vi "MagEncoder_cal_v2.vi"() -> ()   [LabVIEW 2014]
uses:
  <vilib>/eio/EIONode/EIONode.xnode
  <vilib>/rvi/eio/common/nirviEmuTemplateMethod_errors.vi
  <vilib>/rvi/Analysis/measure/butterworth/XNode/niFpgaButterworthFilter.xnode
  <vilib>/rvi/DataTransferAndStorage/Container/XNode/niFpgaContainer.xnode
  <vilib>/rvi/FXPMathLib/FxpSinAndCos/XNode/nifxpmath_SinAndCos.xnode
  <vilib>/rvi/FXPMathLib/FxpSinAndCos/simVIs/DllFxpSinAndCosTemp_sub.vi
  <vilib>/rvi/FXPMathLib/FxpSinAndCos/subVIs/nifxpmath_SinAndCos_SimConfig.ctl
  <vilib>/rvi/interface/RandomDataEmulation/nirviRandomDataFpgaMultiElementTemplate.vi
panel:
  in  "Vy (mm/s)":fxp<+/-,30,6>
  out "Dyr_ramp":fxp<+/-,22,7>
  in  "Dyr_stroke":fxp<+/-,32,7>
  out "Dpr_ramp":fxp<+/-,22,7>
  in  "Dpr_stroke":fxp<+/-,32,7>
  in  "Vp (mm/s)":fxp<+/-,30,6>
  out "omega_p (Mavg w. f)":fxp<+/-,36,18>
  in  "scaled coefficients":i32[](array[numeric])=[946630756, 63555534]
  in  "FIFO":i16(ring) items=["Pitch_F+P", "Yaw_F+P"]
  out "PID (kHz)":fxp<+/-,20,10>
  in  "Set 6":bool
  in  "Set 5":bool
  in  "Set 4":bool
  in  "Set 3":bool
  in  "Set 2":bool
  in  "Set 1":bool
  out "Dy1_d (T)":fxp<+/-,36,13>
  out "omega_y1 (T)":fxp<+/-,36,13>
  out "Dp1_d (T)":fxp<+/-,36,13>
  out "omega_p1 (T)":fxp<+/-,36,13>
  out "Dy2_d (T)":fxp<+/-,36,13>
  out "Dp2_d (T)":fxp<+/-,36,13>
  out "omega_y2 (T)":fxp<+/-,36,13>
  out "omega_p2 (T)":fxp<+/-,36,13>
  out "mt_omega_y2":u32
  out "mt_omega_p2":u32
  out "rad_y2":fxp<+/-,33,20>
  out "D_y2":fxp<+/-,32,7>
  out "rad_y1":fxp<+/-,33,20>
  out "D_y1":fxp<+/-,32,7>
  out "Encoder Position_y1":i32
  out "Encoder Position_y2":i32
  out "Encoder Position_p2":i32
  out "D_p2":fxp<+/-,32,7>
  out "rad_p2":fxp<+/-,33,20>
  out "D_p1":fxp<+/-,32,7>
  out "rad_p1":fxp<+/-,33,20>
  out "Encoder Position_p1":i32
  in  "Mag. factor_y":fxp<+/-,20,3>
  in  "Mag. encoder_y":bool
  out "omega_y (rad/s)":fxp<+/-,36,13>
  out "Dy_d (mm/s)":fxp<+/-,36,13>
  in  "Vy. Est.":i16(ring) items=["T", "Mavg"]
  out "omega_y (Mavg)":fxp<+/-,36,14>
  out "Dy_d (Mavg)":fxp<+/-,36,14>
  in  "Dy_d_M_avg_Tc (uSec)":i32
  out "Dp_d (Mavg)":fxp<+/-,36,14>
  out "omega_p (Mavg)":fxp<+/-,36,14>
  in  "Dp_d_M_avg_Tc (uSec)":i32
  out "Dp_d (T)":fxp<+/-,36,13>
  out "omega_p (T)":fxp<+/-,36,13>
  in  "Vp. Est.":i16(ring) items=["T", "Mavg"]
  in  "Mag. factor_p":fxp<+/-,20,3>
  in  "Mag. encoder_p":bool
  in  "Belt_out_p":fxp<+/-,7,7>
  in  "Belt_in_p":fxp<+/-,6,6>
  in  "Belt_out_y":fxp<+/-,7,7>
  in  "Belt_in_y":fxp<+/-,6,6>
  in  "mt0_omega_p":u32
  in  "Encoder reset":bool
  out "Dpr_sin":fxp<+/-,22,7>
  in  "Sin offset_p":fxp<+/-,22,7>
  in  "Sin magnitude_p":fxp<+/-,21,6>
  out "Dpr_sin_dd":fxp<+/-,35,20>
  out "Dpr_sin_d":fxp<+/-,33,15>
  out "Sin omega_p":fxp<+/-,34,9>
  in  "Sin wave freq._p (Hz)":fxp<+/-,32,6>
  in  "Dpr_step":fxp<+/-,22,7>
  out "Dpr_for":fxp<+/-,22,7>
  in  "Command_p":i16(ring) items=["Step", "Sine", "Ramp"]
  out "Fp_PID":fxp<+/-,36,16>
  in  "Kp_p":fxp<+/-,32,13>
  out "va_p":fxp<+/-,36,7>
  out "vb_p":fxp<+/-,37,8>
  out "vq_p_F":fxp<+/-,20,5> format="%.57g"
  out "vd_p_F":fxp<+/-,20,5>
  in  "Stop motor_p":bool
  out "Dp_d (mm/s)":fxp<+/-,36,13>
  out "omega_p (rad/s)":fxp<+/-,36,13>
  out "mt_omega_p1":u32
  out "rad_p(NrTheta)":fxp<+/-,33,20>
  out "D_p(mm)":fxp<+/-,32,7>
  out "Encoder Position_p":i32
  in  "Encoder reset_p":bool
  out "Dyr_for":fxp<+/-,22,7>
  in  "Command_y":i16(ring) items=["Step", "Sine", "Ramp"]
  out "vb_y":fxp<+/-,38,8>
  out "va_y":fxp<+/-,38,8>
  out "Dyr_sin_dd":fxp<+/-,35,20>
  out "Dyr_sin_d":fxp<+/-,33,15>
  out "Sin omega_y":fxp<+/-,34,9>
  out "Dyr_sin":fxp<+/-,22,7>
  in  "Sin offset_y":fxp<+/-,22,7>
  in  "Sin magnitude_y":fxp<+/-,21,6>
  out "Time now(s)":fxp<+,52,14>
  in  "Sin wave freq._y (Hz)":fxp<+/-,32,6>
  in  "Dyr_step":fxp<+/-,22,7>
  out "Fy_PID":fxp<+/-,36,16>
  in  "Kp_y":fxp<+/-,32,13>
  out "vq_y_F":fxp<+/-,20,5> format="%.57g"
  out "vd_y_F":fxp<+/-,20,5>
  in  "Stop motor_y":bool
  out "Dy_d (T)":fxp<+/-,36,13>
  out "omega_y (T)":fxp<+/-,36,13>
  in  "mt0_omega_y":u32
  out "mt_omega_y1":u32
  out "rad_y(NrTheta)":fxp<+/-,33,20>
  out "D_y(mm)":fxp<+/-,32,7>
  out "Encoder Position_y":i32
  in  "Encoder reset_y":bool
  in  "Ini coe.":bool
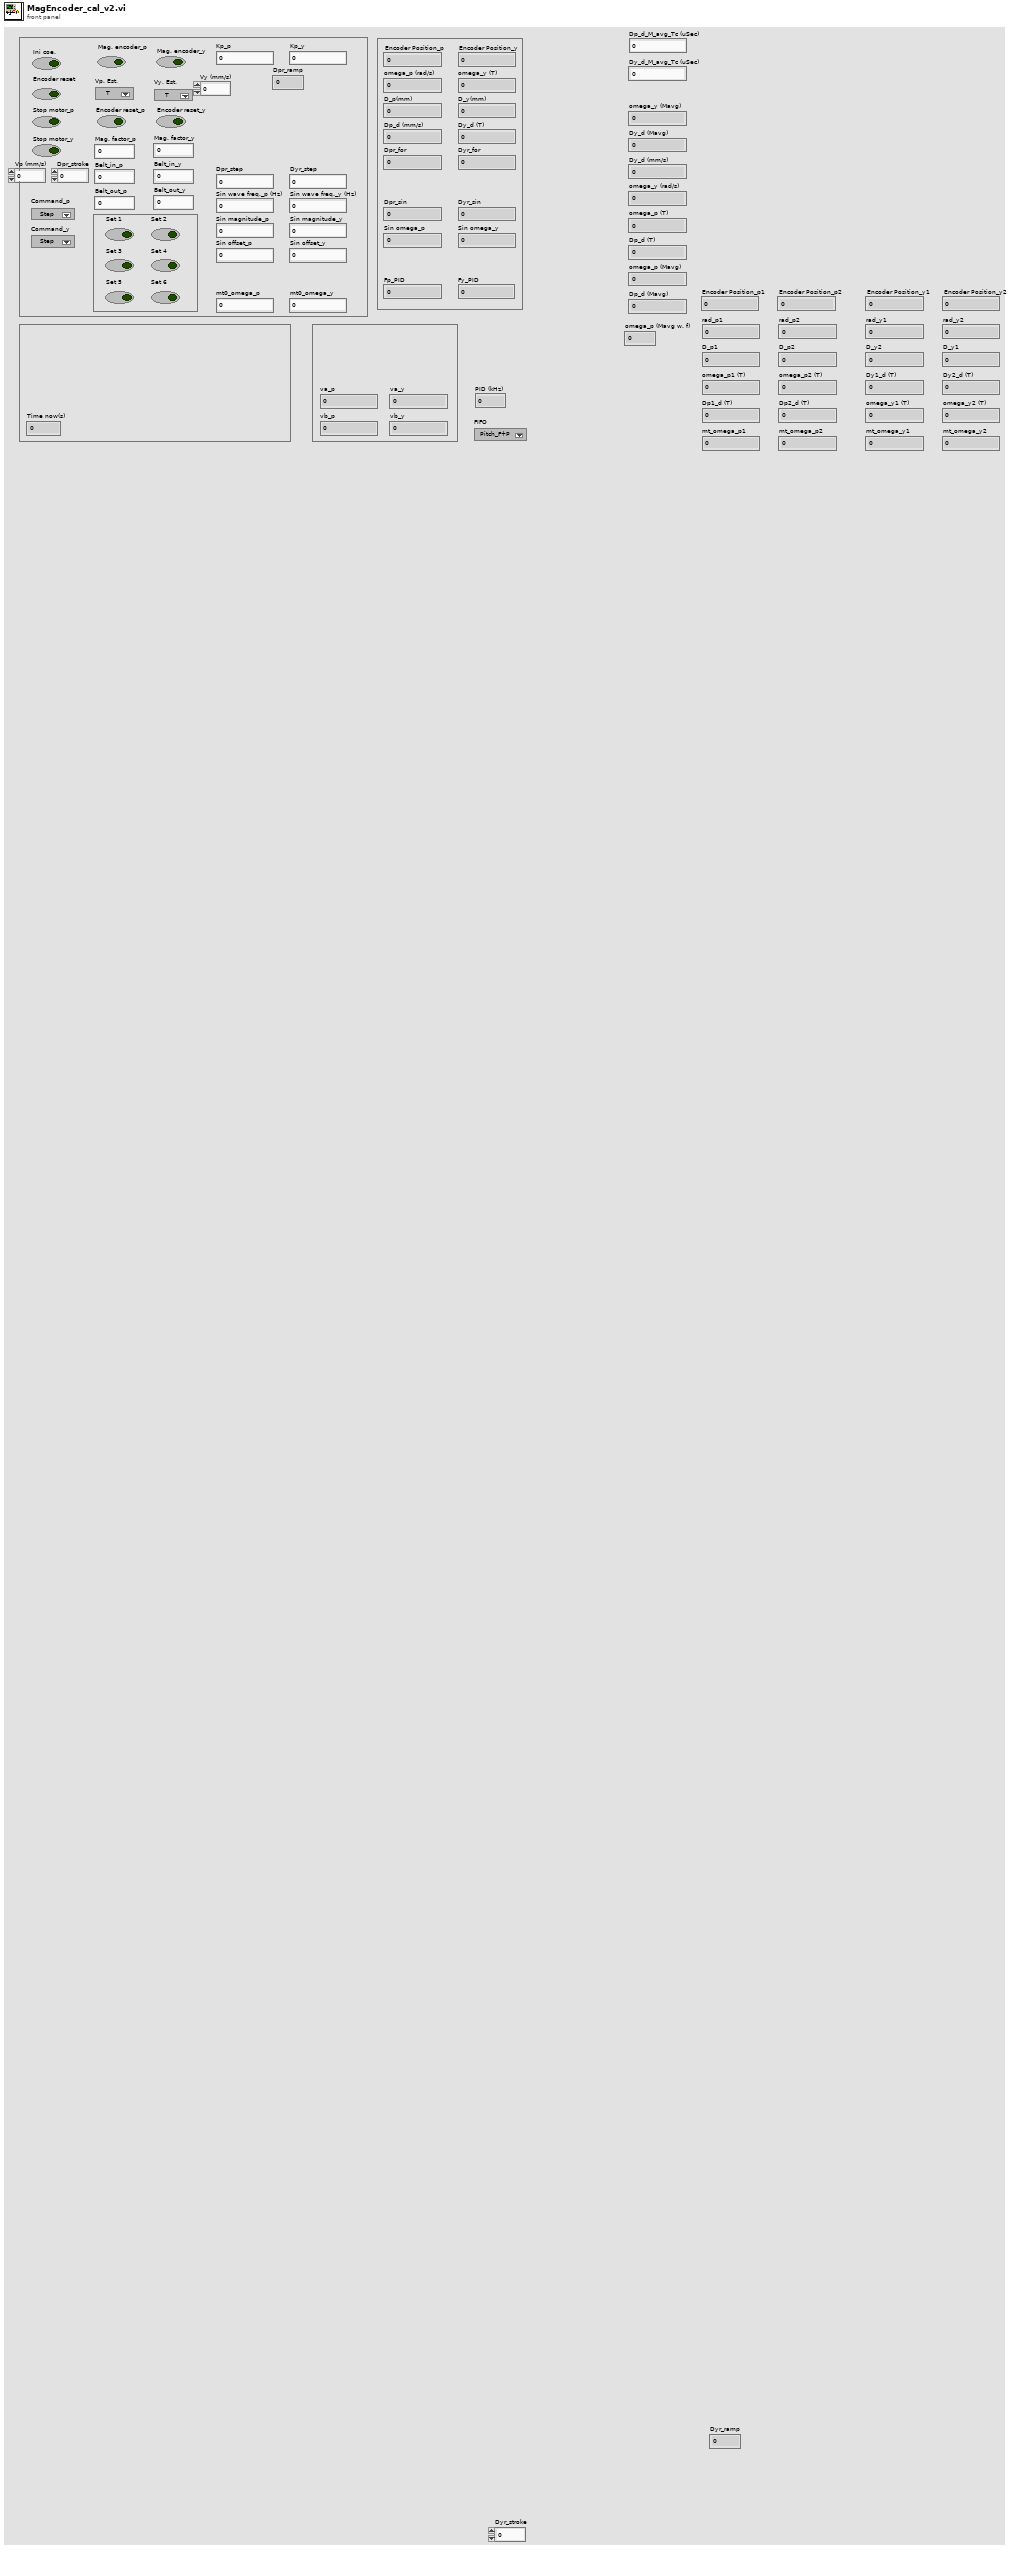
[diagram p1: front panel]
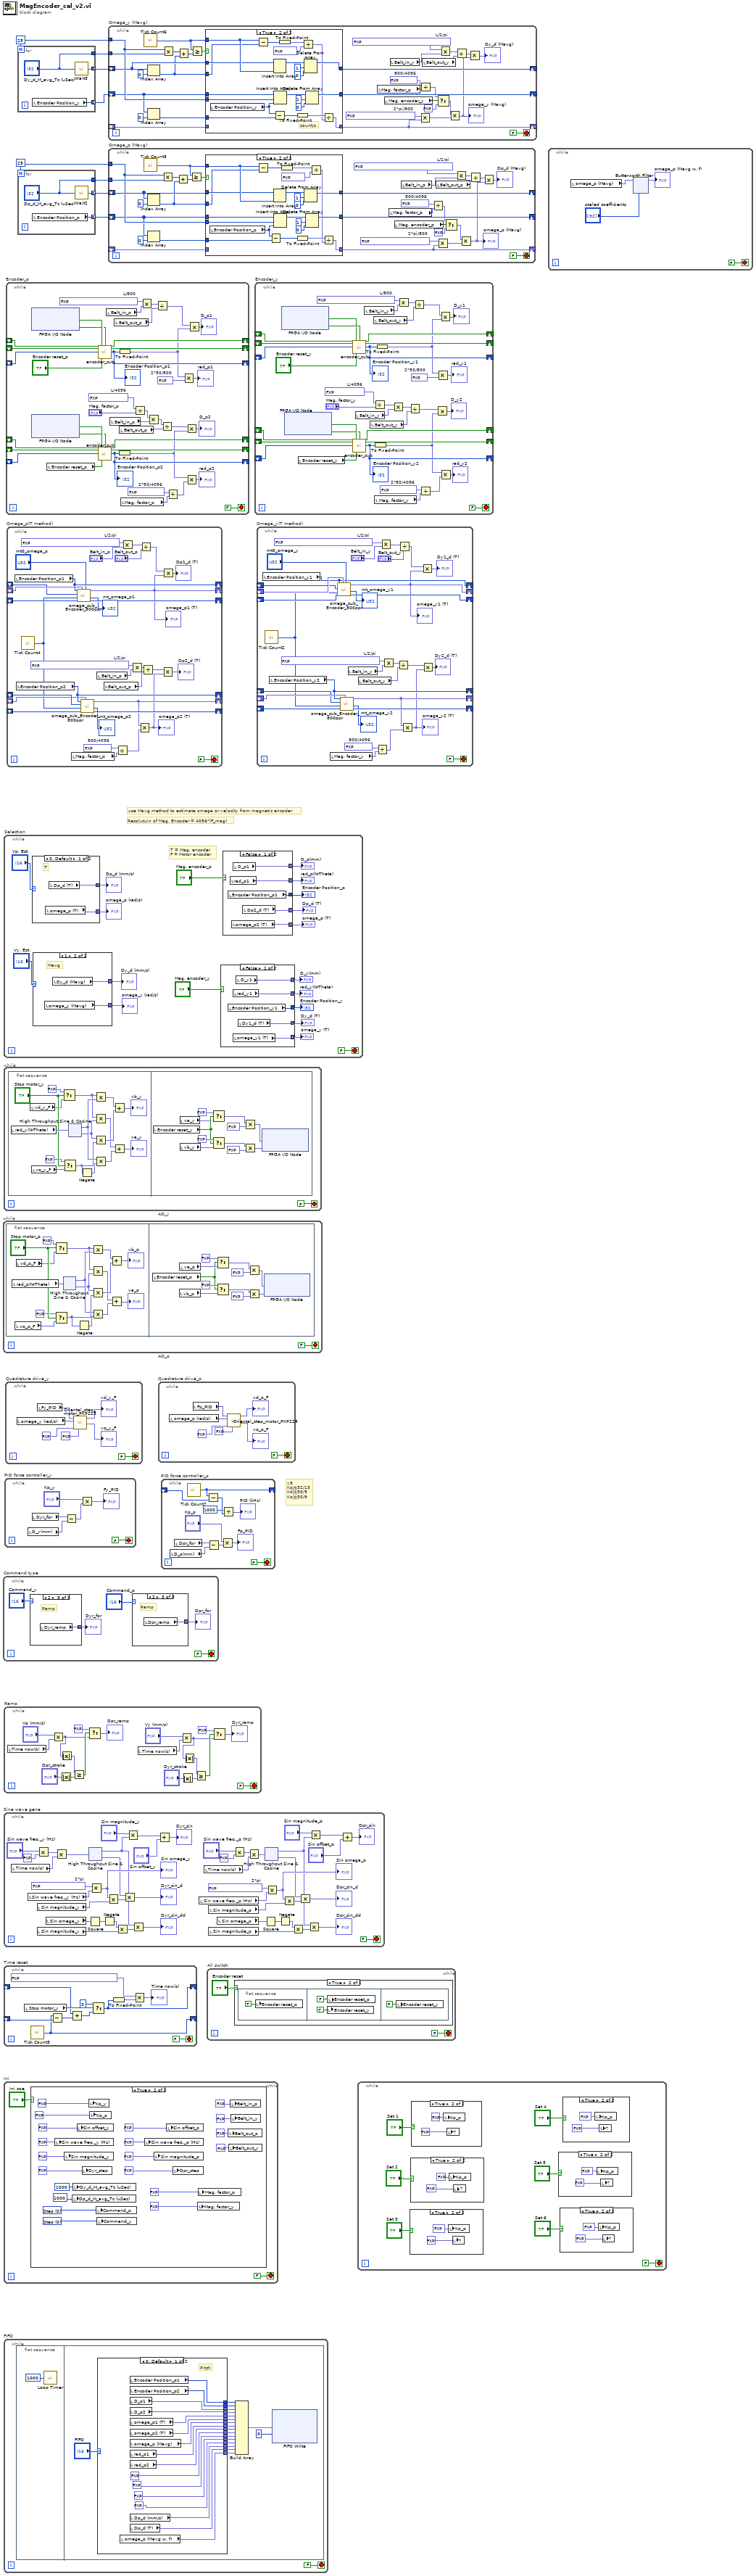
[diagram p0: block diagram]
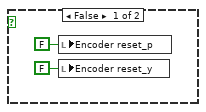
[diagram p10: hidden frame]
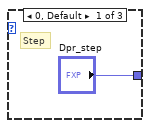
[diagram p11: hidden frame]
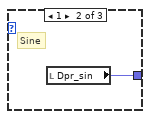
[diagram p12: hidden frame]
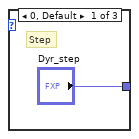
[diagram p13: hidden frame]
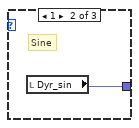
[diagram p14: hidden frame]
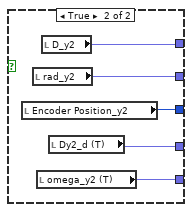
[diagram p15: hidden frame]
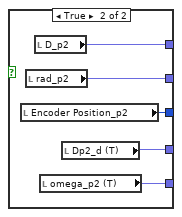
[diagram p16: hidden frame]
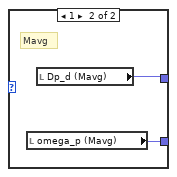
[diagram p17: hidden frame]
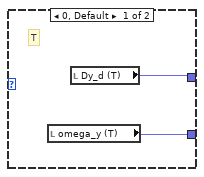
[diagram p18: hidden frame]
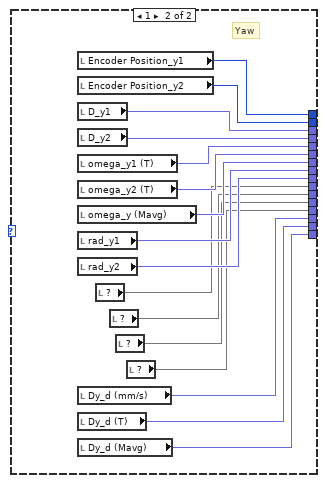
[diagram p20: hidden frame]
diagram:
  w5 = 25
  w8 = 25
  # "v9\nKp改32/13\nKd改30/9\nKo改30/9"
  # "Resolutuin of Mag. Encoder = 4096*(F_mag)"
  # "use Mavg method to estimate omega or velocity from magnetic encoder"
  n1 = while "AO_p" {
    stop <- FALSE stop-if-true
    n2 = flat-sequence {
      frame #0 {
        n3 = local read "rad_p(NrTheta)"() -> (w21:fxp<+/-,33,20>)
        n4 = local read "vq_p_F"() -> (w22:fxp<+/-,20,5>)
        n5 = local read "vd_p_F"() -> (w24:fxp<+/-,20,5>)
        n6 = Select(t=fxp<+/-,20,5> 0.0, s="Stop motor_p", f=w24) -> (s? t:f=w13:fxp<+/-,20,5>)
        n7 = Select(t=fxp<+,1,1> 0.0, s="Stop motor_p", f=w22) -> (s? t:f=w12:fxp<+/-,20,5>)
        n8 = xnode "High Throughput Sine & Cosine"("x (pi)"=w21) -> ("sin(x)"=w15:fxp<+/-,16,2>, "cos(x)"=w14:fxp<+/-,16,2>)
        n9 = Negate(x=w12) -> (-x=w20:fxp<+/-,21,6>)
        n10 = Multiply(x=w13, y=w15) -> (x*y=w19:fxp<+/-,36,7>)
        n11 = Multiply(x=w13, y=w14) -> (x*y=w17:fxp<+/-,36,7>)
        n12 = Multiply(x=w14, y=w12) -> (x*y=w18:fxp<+/-,36,7>)
        n13 = Multiply(x=w15, y=w20) -> (x*y=w16:fxp<+/-,35,6>)
        n14 = Add(x=w19, y=w18) -> (x+y=→"vb_p":fxp<+/-,37,8>)
        n15 = Add(x=w17, y=w16) -> (x+y=→"va_p":fxp<+/-,36,7>)
      }
      frame #1 {
        n16 = local read "Encoder reset_p"() -> (w57:bool)
        n17 = local read "vb_p"() -> (w58:fxp<+/-,37,8>)
        n18 = local read "va_p"() -> (w59:fxp<+/-,36,7>)
        n19 = Select(t=fxp<+,2,2> 3.0, s=w57, f=w59) -> (s? t:f=w65:fxp<+/-,36,7>)
        n20 = Select(t=fxp<+,1,1> 0.0, s=w57, f=w58) -> (s? t:f=w64:fxp<+/-,37,8>)
        n21 = Multiply(x=w65, y=fxp<+/-,1,0> -0.5) -> (x*y=w60:fxp<+/-,36,6>)
        n22 = Multiply(x=w64, y=fxp<+/-,1,0> -0.5) -> (x*y=w61:fxp<+/-,36,6>)
        n23 = xnode "FPGA I/O Node"("Mod8/AO0"=w60, "Mod8/AO1"=w61) -> ()  [unwired: 2 in, 2 out]
      }
    }
  }
  n24 = while "Command type" {
    stop <- FALSE stop-if-true
    n25 = case shown="2" "Command_y" {
      tunnel: ["Dyr_step" w77 w78] -> w71
      frame 0, Default {
        # "Step"
      }
      frame 1 {
        # "Sine"
        n26 = local read "Dyr_sin"() -> (w77:fxp<+/-,22,7>)
      }
      frame 2 {
        # "Ramp"
        n27 = local read "Dyr_ramp"() -> (w78:fxp<+/-,22,7>)
      }
    }
    "Dyr_for" <- w71
    n28 = case shown="2" "Command_p" {
      tunnel: ["Dpr_step" w74 w75] -> w69
      frame 0, Default {
        # "Step"
      }
      frame 1 {
        # "Sine"
        n29 = local read "Dpr_sin"() -> (w74:fxp<+/-,22,7>)
      }
      frame 2 {
        # "Ramp"
        n30 = local read "Dpr_ramp"() -> (w75:fxp<+/-,22,7>)
      }
    }
    "Dpr_for" <- w69
  }
  n31 = while "AO_y" {
    stop <- FALSE stop-if-true
    n32 = flat-sequence {
      frame #0 {
        n33 = local read "rad_y(NrTheta)"() -> (w96:fxp<+/-,33,20>)
        n34 = local read "vd_y_F"() -> (w94:fxp<+/-,20,5>)
        n35 = local read "vq_y_F"() -> (w93:fxp<+/-,20,5>)
        n36 = Select(t=fxp<+/-,20,5> 0.0, s="Stop motor_y", f=w94) -> (s? t:f=w88:fxp<+/-,20,5>)
        n37 = Select(t=fxp<+/-,20,5> 0.0, s="Stop motor_y", f=w93) -> (s? t:f=w87:fxp<+/-,20,5>)
        n38 = xnode "High Throughput Sine & Cosine"("x (pi)"=w96) -> ("sin(x)"=w90:fxp<+/-,17,2>, "cos(x)"=w89:fxp<+/-,17,2>)
        n39 = Negate(x=w87) -> (-x=w86:fxp<+/-,21,6>)
        n40 = Multiply(x=w88, y=w90) -> (x*y=w85:fxp<+/-,37,7>)
        n41 = Multiply(x=w88, y=w89) -> (x*y=w83:fxp<+/-,37,7>)
        n42 = Multiply(x=w89, y=w87) -> (x*y=w84:fxp<+/-,37,7>)
        n43 = Multiply(x=w90, y=w86) -> (x*y=w82:fxp<+/-,36,6>)
        n44 = Add(x=w85, y=w84) -> (x+y=→"vb_y":fxp<+/-,38,8>)
        n45 = Add(x=w83, y=w82) -> (x+y=→"va_y":fxp<+/-,37,7>)
      }
      frame #1 {
        n46 = local read "Encoder reset_y"() -> (w129:bool)
        n47 = local read "va_y"() -> (w128:fxp<+/-,38,8>)
        n48 = local read "vb_y"() -> (w127:fxp<+/-,38,8>)
        n49 = Select(t=fxp<+,2,2> 3.0, s=w129, f=w128) -> (s? t:f=w133:fxp<+/-,38,8>)
        n50 = Select(t=fxp<+,1,1> 0.0, s=w129, f=w127) -> (s? t:f=w132:fxp<+/-,38,8>)
        n51 = Multiply(x=w133, y=fxp<+/-,1,0> -0.5) -> (x*y=w136:fxp<+/-,39,8>)
        n52 = Multiply(x=w132, y=fxp<+/-,1,0> -0.5) -> (x*y=w137:fxp<+/-,37,6>)
        n53 = xnode "FPGA I/O Node"("Mod8/AO2"=w136, "Mod8/AO3"=w137) -> ()  [unwired: 2 in, 2 out]
      }
    }
  }
  n54 = while "Sine wave gene" {
    stop <- FALSE stop-if-true
    w143 = fxp<+,20,3> 6.2831878662109375  # 2*pi
    w175 = fxp<+,20,3> 6.2831878662109375  # 2*pi
    n55 = local read "Time now(s)"() -> (w181:fxp<+,52,14>)
    n56 = local read "Sin wave freq._y (Hz)"() -> (w174:fxp<+/-,32,6>)
    n57 = Multiply(x="Sin wave freq._y (Hz)", y=fxp<+/-,10,3> 2.0) -> (x*y=w182:fxp<+/-,41,9>)
    n58 = local read "Sin magnitude_y"() -> (w172:fxp<+/-,21,6>)
    n59 = local read "Sin magnitude_y"() -> (w165:fxp<+/-,21,6>)
    n60 = local read "Sin omega_y"() -> (w168:fxp<+/-,34,9>)
    n61 = Multiply(x=w182, y=w181) -> (x*y=w180:fxp<+/-,41,19>)
    n62 = Square(x=w168) -> (x^2=w167:fxp<+,34,18>)
    n63 = xnode "High Throughput Sine & Cosine"("x (pi)"=w180) -> ("sin(x)"=w162:fxp<+/-,16,2>, "cos(x)"=w170:fxp<+/-,16,2>)
    n64 = Multiply(x=w175, y=w174) -> (x*y=w173:fxp<+/-,34,9>)
    "Sin omega_y" <- w173
    n65 = Negate(x=w167) -> (-x=w166:fxp<+/-,35,19>)
    n66 = Multiply(x=w173, y=w172) -> (x*y=w171:fxp<+/-,33,15>)
    n67 = Multiply(x=w166, y=w165) -> (x*y=w164:fxp<+/-,34,20>)
    n68 = Multiply(x=w170, y=w171) -> (x*y=→"Dyr_sin_d":fxp<+/-,33,15>)
    n69 = Multiply(x="Sin magnitude_y", y=w162) -> (x*y=w178:fxp<+/-,37,8>)
    n70 = Multiply(x=w162, y=w164) -> (x*y=→"Dyr_sin_dd":fxp<+/-,35,20>)
    n71 = Add(x=w178, y="Sin offset_y") -> (x+y=→"Dyr_sin":fxp<+/-,37,8>)
    n72 = local read "Sin wave freq._p (Hz)"() -> (w139:fxp<+/-,32,6>)
    n73 = local read "Time now(s)"() -> (w157:fxp<+,52,14>)
    n74 = local read "Sin magnitude_p"() -> (w140:fxp<+/-,21,6>)
    n75 = local read "Sin magnitude_p"() -> (w142:fxp<+/-,21,6>)
    n76 = local read "Sin omega_p"() -> (w141:fxp<+/-,34,9>)
    n77 = Multiply(x="Sin wave freq._p (Hz)", y=fxp<+/-,10,3> 2.0) -> (x*y=w161:fxp<+/-,42,9>)
    n78 = Multiply(x=w161, y=w157) -> (x*y=w158:fxp<+/-,41,19>)
    n79 = Square(x=w141) -> (x^2=w153:fxp<+,34,18>)
    n80 = xnode "High Throughput Sine & Cosine"("x (pi)"=w158) -> ("sin(x)"=w144:fxp<+/-,16,2>, "cos(x)"=w149:fxp<+/-,16,2>)
    n81 = Multiply(x=w143, y=w139) -> (x*y=w156:fxp<+/-,34,9>)
    "Sin omega_p" <- w156
    n82 = Negate(x=w153) -> (-x=w152:fxp<+/-,35,19>)
    n83 = Multiply(x=w156, y=w140) -> (x*y=w155:fxp<+/-,33,15>)
    n84 = Multiply(x=w152, y=w142) -> (x*y=w151:fxp<+/-,35,19>)
    n85 = Multiply(x=w149, y=w155) -> (x*y=→"Dpr_sin_d":fxp<+/-,33,15>)
    n86 = Multiply(x=w144, y=w151) -> (x*y=→"Dpr_sin_dd":fxp<+/-,35,20>)
    n87 = Multiply(x="Sin magnitude_p", y=w144) -> (x*y=w147:fxp<+/-,37,8>)
    n88 = Add(x=w147, y="Sin offset_p") -> (x+y=→"Dpr_sin":fxp<+/-,37,8>)
  }
  n89 = while "Time reset" {
    shift-right: [w254] -> _
    shift-left: _ -> [w255]
    shift-right: [w249] -> _
    shift-left: _ -> [w250]
    stop <- FALSE stop-if-true
    n90 = local read "Stop motor_y"() -> (w256:bool)
    n91 = call "Tick Count3"() -> ("Tick Count(uSec)"=w254:u32)
    n92 = Subtract(x=w254, y=w255) -> (x-y=w253:u32)
    n93 = Add(x=w250, y=w253) -> (x+y=w252:u32)
    n94 = Select(t=u32 0, s=w256, f=w252) -> (s? t:f=w249:u32)
    n95 = To Fixed-Point(number=w249) -> (fixed-point=w248:fxp<+,32,32>)  [unwired: 1 in]
    n96 = Multiply(x=fxp<+,20,-18> 1.0000003385357559e-06, y=w248) -> (x*y=→"Time now(s)":fxp<+,52,14>)
  }
  n97 = while "Ini" {
    stop <- FALSE stop-if-true
    n98 = case shown="True" "Ini coe." {
      frame False {
      }
      frame True {
        w272 = i16 0 items=["Step", "Sine"] ("Command_p")
        w273 = i16 0 items=["Step", "Sine"] ("Command_y")
        n99 = local write "Sin wave freq._y (Hz)"(fxp<+/-,32,6> 1.0 ("Sin wave freq. (Hz)")) -> ()
        n100 = local write "Sin magnitude_y"(fxp<+/-,22,7> 5.0 ("Sin magnitude")) -> ()
        n101 = local write "Dp_d_M_avg_Tc (uSec)"(u32 1000 ("D_d_M_avg_Tc (uSec)")) -> ()
        n102 = local write "Dy_d_M_avg_Tc (uSec)"(1000 ("Dy_d_M_avg_Tc (uSec)")) -> ()
        n103 = local write "Sin offset_y"(fxp<+/-,38,9> 0.0 ("Sin offset")) -> ()
        n104 = local write "Dyr_step"(fxp<+/-,22,7> 0.0 ("Dr")) -> ()
        n105 = local write "Kp_y"(fxp<+/-,36,9> 30.0 ("Kp")) -> ()
        n106 = local write "Kp_p"(fxp<+/-,36,9> 30.0 ("Kp_p")) -> ()
        n107 = local write "Command_p"(w272) -> ()
        n108 = local write "Command_y"(w273) -> ()
        n109 = local write "Sin wave freq._p (Hz)"(fxp<+/-,32,6> 1.0 ("Sin wave freq._p (Hz)")) -> ()
        n110 = local write "Sin magnitude_p"(fxp<+/-,21,6> 5.0 ("Sin magnitude_p")) -> ()
        n111 = local write "Sin offset_p"(fxp<+/-,22,7> 0.0 ("Sin offset_p")) -> ()
        n112 = local write "Dpr_step"(fxp<+/-,22,7> 0.0 ("Dpr_step")) -> ()
        n113 = local write "Mag. factor_y"(fxp<+/-,36,9> 1.0 ("Kd_p")) -> ()
        n114 = local write "Mag. factor_p"(fxp<+/-,36,9> 1.0 ("Ki_p")) -> ()
        n115 = local write "Belt_out_p"(fxp<+/-,7,7> 22.0 ("Belt_op")) -> ()
        n116 = local write "Belt_out_y"(fxp<+/-,7,7> 22.0 ("Belt_oy")) -> ()
        n117 = local write "Belt_in_p"(fxp<+/-,6,6> 16.0 ("Belt_mp")) -> ()
        n118 = local write "Belt_in_y"(fxp<+/-,6,6> 16.0 ("Belt_my")) -> ()
      }
    }
  }
  n119 = while "FIFO" {
    stop <- FALSE stop-if-true
    n120 = flat-sequence {
      frame #0 {
        n121 = call "Loop Timer"("Count(uSec)"=u32 1000) -> ()  [unwired: 1 out]
      }
      frame #1 {
        n122 = case shown="0, Default" "FIFO" {
          tunnel: [w315 w331] -> w299
          tunnel: [w314 w330] -> w298
          tunnel: [w313 w329] -> w297
          tunnel: [w312 w328] -> w296
          tunnel: [w309 w325] -> w294
          tunnel: [w310 w326] -> w293
          tunnel: [w311 w327] -> w292
          tunnel: [w307 w323] -> w291
          tunnel: [fxp<+,1,1> 0.0 w322] -> w290
          tunnel: [fxp<+,1,1> 0.0 w321] -> w289
          tunnel: [fxp<+,1,1> 0.0 w320] -> w288
          tunnel: [fxp<+,1,1> 0.0 w319] -> w287
          tunnel: [w306 w318] -> w286
          tunnel: [w305 w317] -> w285
          tunnel: [w304 w316] -> w284
          tunnel: [w308 w324] -> w282
          frame 0, Default {
            # "Pitch"
            n123 = local read "omega_p (Mavg w. f)"() -> (w304:fxp<+/-,36,18>)
            n124 = local read "Encoder Position_p1"() -> (w315:i32)
            n125 = local read "Encoder Position_p2"() -> (w314:i32)
            n126 = local read "D_p1"() -> (w313:fxp<+/-,32,7>)
            n127 = local read "D_p2"() -> (w312:fxp<+/-,32,7>)
            n128 = local read "omega_p1 (T)"() -> (w311:fxp<+/-,36,13>)
            n129 = local read "omega_p2 (T)"() -> (w310:fxp<+/-,36,13>)
            n130 = local read "omega_p (Mavg)"() -> (w309:fxp<+/-,36,14>)
            n131 = local read "rad_p1"() -> (w308:fxp<+/-,33,20>)
            n132 = local read "rad_p2"() -> (w307:fxp<+/-,33,20>)
            n133 = local read "Dp_d (mm/s)"() -> (w306:fxp<+/-,36,13>)
            n134 = local read "Dp_d (T)"() -> (w305:fxp<+/-,36,13>)
          }
          frame 1 {
            # "Yaw"
            n135 = local read "Encoder Position_y1"() -> (w331:i32)
            n136 = local read "Encoder Position_y2"() -> (w330:i32)
            n137 = local read "D_y1"() -> (w329:fxp<+/-,32,7>)
            n138 = local read "D_y2"() -> (w328:fxp<+/-,32,7>)
            n139 = local read "omega_y1 (T)"() -> (w327:fxp<+/-,36,13>)
            n140 = local read "omega_y2 (T)"() -> (w326:fxp<+/-,36,13>)
            n141 = local read "omega_y (Mavg)"() -> (w325:fxp<+/-,36,14>)
            n142 = local read "rad_y1"() -> (w324:fxp<+/-,33,20>)
            n143 = local read "rad_y2"() -> (w323:fxp<+/-,33,20>)
            n144 = local read "Dy_d (mm/s)"() -> (w318:fxp<+/-,36,13>)
            n145 = local read "Dy_d (T)"() -> (w317:fxp<+/-,36,13>)
            n146 = local read "Dy_d (Mavg)"() -> (w316:fxp<+/-,36,14>)
            n147 = local read item#-1() -> (w322)
            n148 = local read item#-1() -> (w321)
            n149 = local read item#-1() -> (w320)
            n150 = local read item#-1() -> (w319)
          }
        }
        n151 = Build Array(w299, w298, w297, w296, w292, w293, w294, w282, w291, w290, w289, w288, w287, w286, w285, w284) -> (w283:fxp<+/-,57,32>[])
        n152 = xnode ("FIFO Write")("Element"=w283, "Timeout"=0) -> ()  [unwired: 1 in, 2 out]
      }
    }
  }
  n153 = while "Selection" {
    stop <- FALSE stop-if-true
    # "T = Mag. encoder\nF = Motor encoder"
    n154 = case shown="0, Default" "Vp. Est." {
      tunnel: [w372 w373] -> w346
      tunnel: [w371 w374] -> w347
      frame 0, Default {
        # "T"
        n155 = local read "omega_p (T)"() -> (w372:fxp<+/-,36,13>)
        n156 = local read "Dp_d (T)"() -> (w371:fxp<+/-,36,13>)
      }
      frame 1 {
        # "Mavg"
        n157 = local read "omega_p (Mavg)"() -> (w373:fxp<+/-,36,14>)
        n158 = local read "Dp_d (Mavg)"() -> (w374:fxp<+/-,36,14>)
      }
    }
    "Dp_d (mm/s)" <- w347
    "omega_p (rad/s)" <- w346
    n159 = case shown="1" "Vy. Est." {
      tunnel: [w376 w378] -> w349
      tunnel: [w375 w377] -> w350
      frame 0, Default {
        # "T"
        n160 = local read "omega_y (T)"() -> (w375:fxp<+/-,36,13>)
        n161 = local read "Dy_d (T)"() -> (w376:fxp<+/-,36,13>)
      }
      frame 1 {
        # "Mavg"
        n162 = local read "omega_y (Mavg)"() -> (w377:fxp<+/-,36,14>)
        n163 = local read "Dy_d (Mavg)"() -> (w378:fxp<+/-,36,14>)
      }
    }
    "Dy_d (mm/s)" <- w349
    "omega_y (rad/s)" <- w350
    n164 = case shown="False" "Mag. encoder_y" {
      tunnel: [w355 w359] -> w337
      tunnel: [w354 w360] -> w338
      tunnel: [w353 w358] -> w340
      tunnel: [w351 w357] -> w334
      tunnel: [w352 w356] -> w333
      frame False {
        n165 = local read "Encoder Position_y1"() -> (w353:i32)
        n166 = local read "rad_y1"() -> (w355:fxp<+/-,33,20>)
        n167 = local read "omega_y1 (T)"() -> (w351:fxp<+/-,36,13>)
        n168 = local read "D_y1"() -> (w354:fxp<+/-,32,7>)
        n169 = local read "Dy1_d (T)"() -> (w352:fxp<+/-,36,13>)
      }
      frame True {
        n170 = local read "Encoder Position_y2"() -> (w358:i32)
        n171 = local read "rad_y2"() -> (w359:fxp<+/-,33,20>)
        n172 = local read "omega_y2 (T)"() -> (w357:fxp<+/-,36,13>)
        n173 = local read "D_y2"() -> (w360:fxp<+/-,32,7>)
        n174 = local read "Dy2_d (T)"() -> (w356:fxp<+/-,36,13>)
      }
    }
    "D_y(mm)" <- w338
    "rad_y(NrTheta)" <- w337
    "Encoder Position_y" <- w340
    "Dy_d (T)" <- w333
    "omega_y (T)" <- w334
    n175 = case shown="False" "Mag. encoder_p" {
      tunnel: [w365 w370] -> w342
      tunnel: [w364 w369] -> w343
      tunnel: [w363 w368] -> w344
      tunnel: [w361 w367] -> w336
      tunnel: [w362 w366] -> w335
      frame False {
        n176 = local read "Encoder Position_p1"() -> (w363:i32)
        n177 = local read "rad_p1"() -> (w364:fxp<+/-,33,20>)
        n178 = local read "omega_p2 (T)"() -> (w361:fxp<+/-,36,13>)
        n179 = local read "D_p1"() -> (w365:fxp<+/-,32,7>)
        n180 = local read "Dp2_d (T)"() -> (w362:fxp<+/-,36,13>)
      }
      frame True {
        n181 = local read "Encoder Position_p2"() -> (w368:i32)
        n182 = local read "rad_p2"() -> (w369:fxp<+/-,33,20>)
        n183 = local read "D_p2"() -> (w370:fxp<+/-,32,7>)
        n184 = local read "omega_p2 (T)"() -> (w367:fxp<+/-,36,13>)
        n185 = local read "Dp2_d (T)"() -> (w366:fxp<+/-,36,13>)
      }
    }
    "D_p(mm)" <- w342
    "rad_p(NrTheta)" <- w343
    "Encoder Position_p" <- w344
    "Dp_d (T)" <- w335
    "omega_p (T)" <- w336
  }
  n186 = while "Ramp" {
    stop <- FALSE stop-if-true
    n187 = local read "Time now(s)"() -> (w396:fxp<+,52,14>)
    n188 = Multiply(x="Vp (mm/s)", y=w396) -> (x*y=w383:fxp<+/-,64,20>)
    n189 = Absolute Value(x="Dpr_stroke") -> (abs(x)=w385:fxp<+,32,7>)
    n190 = Absolute Value(x=w383) -> (abs(x)=w384:fxp<+,64,20>)
    n191 = Greater Or Equal?(x=w384, y=w385) -> (x >= y?=w395:bool)
    n192 = Select(t=fxp<+/-,64,46> 0.0, s=w395, f=w383) -> (s? t:f=→"Dpr_ramp":fxp<+/-,64,46>)
    n193 = local read "Time now(s)"() -> (w389:fxp<+,52,14>)
    n194 = Multiply(x="Vy (mm/s)", y=w389) -> (x*y=w379:fxp<+/-,64,20>)
    n195 = Absolute Value(x="Dyr_stroke") -> (abs(x)=w381:fxp<+,32,7>)
    n196 = Absolute Value(x=w379) -> (abs(x)=w380:fxp<+,64,20>)
    n197 = Greater Or Equal?(x=w380, y=w381) -> (x >= y?=w392:bool)
    n198 = Select(t=fxp<+/-,64,46> 0.0, s=w392, f=w379) -> (s? t:f=→"Dyr_ramp":fxp<+/-,64,46>)
  }
  n199 = while "PID force controller_y" {
    stop <- FALSE stop-if-true
    n200 = local read "D_y(mm)"() -> (w401:fxp<+/-,32,7>)
    n201 = local read "Dyr_for"() -> (w402:fxp<+/-,22,7>)
    n202 = Subtract(x=w402, y=w401) -> (x-y=w400:fxp<+/-,33,8>)
    n203 = Multiply(x="Kp_y", y=w400) -> (x*y=→"Fy_PID":fxp<+/-,64,20>)
  }
  n204 = while "Quadrature drive_y" {
    stop <- FALSE stop-if-true
    n205 = local read "omega_y (rad/s)"() -> (w410:fxp<+/-,36,13>)
    n206 = local read "Fy_PID"() -> (w406:fxp<+/-,36,16>)
    n207 = call "Oriental_step_motor_PKP225.vi"("F_Threshold"=fxp<+,12,12> 10.0, "dFmr"=fxp<+/-,25,15> 0.0, "omega"=w410, "Fmr"=w406) -> ("vq_F"=→"vq_y_F":fxp<+/-,20,5>, "vd_F"=→"vd_y_F":fxp<+/-,20,5>)  [unwired: 6 in]
  }
  n208 = while "Encoder_p" {
    shift-right: [w448] -> _
    shift-left: _ -> [w447]
    shift-right: [w449] -> _
    shift-left: _ -> [w446]
    shift-right: [w443] -> _
    shift-left: _ -> [w445]
    shift-right: [w434] -> _
    shift-left: _ -> [w433]
    shift-right: [w435] -> _
    shift-left: _ -> [w436]
    shift-right: [w430] -> _
    shift-left: _ -> [w431]
    stop <- FALSE stop-if-true
    w426 = fxp<+/-,20,-5> 0.00048828125  # L/4096
    w424 = fxp<+/-,16,1> 0.0244140625  # 2*50/4096
    w442 = fxp<+/-,20,-5> 0.002499997615814209  # L/800
    w416 = fxp<+/-,16,1> 0.125  # 2*50/800
    n209 = xnode "FPGA I/O Node"() -> ("Mod7/DIO0"=w451:bool, "Mod7/DIO1"=w450:bool)  [unwired: 2 in, 2 out]
    n210 = xnode "FPGA I/O Node"() -> ("Mod7/DIO4"=w438:bool, "Mod7/DIO5"=w437:bool)  [unwired: 2 in, 2 out]
    n211 = local read "Encoder reset_p"() -> (w432:bool)
    n212 = call "encoder_sub.vi"("A_pre"=w447, "B_pre"=w446, "Encoder Position_pre"=w445, "A input"=w451, "Encoder Position Reset"="Encoder reset_p", "B input"=w450) -> ("A"=w448:bool, "B"=w449:bool, "Encoder Position (Counts)"=w443:i32)  [unwired: 19 in]
    "Encoder Position_p1" <- w443
    n213 = call "encoder_sub.vi"("A_pre"=w433, "B_pre"=w436, "Encoder Position_pre"=w431, "A input"=w438, "Encoder Position Reset"=w432, "B input"=w437) -> ("A"=w434:bool, "B"=w435:bool, "Encoder Position (Counts)"=w430:i32)  [unwired: 19 in]
    "Encoder Position_p2" <- w430
    n214 = local read "Belt_in_p"() -> (w441:fxp<+/-,6,6>)
    n215 = local read "Belt_in_p"() -> (w427:fxp<+/-,6,6>)
    n216 = local read "Belt_out_p"() -> (w439:fxp<+/-,7,7>)
    n217 = To Fixed-Point(number=w430) -> (fixed-point=w412:fxp<+/-,32,32>)  [unwired: 1 in]
    n218 = To Fixed-Point(number=w443) -> (fixed-point=w417:fxp<+/-,32,32>)  [unwired: 1 in]
    n219 = local read "Belt_out_p"() -> (w429:fxp<+/-,7,7>)
    n220 = local read "Mag. factor_p"() -> (w423:fxp<+/-,20,3>)
    n221 = Divide(x=w426, y="Mag. factor_p") -> (x/y=w425:fxp<+/-,41,13>)
    n222 = Multiply(x=w442, y=w441) -> (x*y=w440:fxp<+/-,26,1>)
    n223 = Multiply(x=w425, y=w427) -> (x*y=w428:fxp<+/-,46,18>)
    n224 = Divide(x=w440, y=w439) -> (x/y=w419:fxp<+/-,33,1>)
    n225 = Divide(x=w428, y=w429) -> (x/y=w414:fxp<+/-,53,18>)
    n226 = Divide(x=w424, y=w423) -> (x/y=w411:fxp<+/-,32,1>)
    n227 = Multiply(x=w417, y=w416) -> (x*y=→"rad_p1":fxp<+/-,33,20>)
    n228 = Multiply(x=w414, y=w412) -> (x*y=→"D_p2":fxp<+/-,37,7>)
    n229 = Multiply(x=w412, y=w411) -> (x*y=→"rad_p2":fxp<+/-,33,20>)
    n230 = Multiply(x=w419, y=w417) -> (x*y=→"D_p1":fxp<+/-,32,7>)
  }
  n231 = while "Omega_p(T method)" {
    shift-right: [w484] -> _
    shift-left: _ -> [w482]
    shift-right: [w455] -> _
    shift-left: _ -> [w483]
    shift-right: [w480] -> _
    shift-left: _ -> [w481]
    shift-right: [w471] -> _
    shift-left: _ -> [w470]
    shift-right: [w464] -> _
    shift-left: _ -> [w469]
    shift-right: [w468] -> _
    shift-left: _ -> [w467]
    stop <- FALSE stop-if-true
    w462 = fxp<+/-,32,0> 0.3183098859153688  # L/2/pi
    w473 = fxp<+,32,0> 0.1953125  # 800/4096
    w477 = fxp<+/-,32,0> 0.3183098859153688  # L/2/pi
    n232 = local read "Encoder Position_p1"() -> (w484:i32)
    n233 = local read "Encoder Position_p2"() -> (w471:i32)
    n234 = call "Tick Count4"() -> ("Tick Count(Ticks)"=w466:u32)
    n235 = local read "Mag. factor_p"() -> (w472:fxp<+/-,20,3>)
    n236 = call "omega_sub_Encoder_800ppr.vi"("mt0"="mt0_omega_p", "omega_pre"=w483, "ticks_m_pre"=w481, "ticks"=w466, "count_pre"=w482, "count"=w484) -> ("ticks_m"=w480:u32, "mt"=→"mt_omega_p1":u32, "omega"=w455:fxp<+/-,36,13>)  [unwired: 3 in]
    "omega_p1 (T)" <- w455
    n237 = call "omega_sub_Encoder_800ppr.vi"("omega_pre"=w469, "ticks_m_pre"=w467, "ticks"=w466, "count_pre"=w470, "count"=w471) -> ("ticks_m"=w468:u32, "mt"=→"mt_omega_p2":u32, "omega"=w464:fxp<+/-,36,13>)  [unwired: 4 in]
    n238 = local read "Belt_in_p"() -> (w460:fxp<+/-,6,6>)
    n239 = local read "Belt_out_p"() -> (w459:fxp<+/-,7,7>)
    n240 = Divide(x=w473, y=w472) -> (x/y=w463:fxp<+/-,32,1>)
    n241 = Multiply(x=w477, y="Belt_in_p") -> (x*y=w475:fxp<+/-,38,6>)
    n242 = Multiply(x=w462, y=w460) -> (x*y=w461:fxp<+/-,38,6>)
    n243 = Multiply(x=w464, y=w463) -> (x*y=w453:fxp<+/-,36,13>)
    "omega_p2 (T)" <- w453
    n244 = Divide(x=w475, y="Belt_out_p") -> (x/y=w456:fxp<+/-,20,1>)
    n245 = Divide(x=w461, y=w459) -> (x/y=w454:fxp<+/-,45,6>)
    n246 = Multiply(x=w454, y=w453) -> (x*y=→"Dp2_d (T)":fxp<+/-,36,13>)
    n247 = Multiply(x=w456, y=w455) -> (x*y=→"Dp1_d (T)":fxp<+/-,36,13>)
  }
  n248 = for {
    N: w5 -> [_]
    tunnel: [w487] -> w4 mode=indexing
    tunnel: [w486] -> w3 mode=indexing
    tunnel: ["Dy_d_M_avg_Tc (uSec)"] -> w2
    n249 = local read "Encoder Position_y"() -> (w486:i32)
    n250 = call "Wait3"("Count(uSec)"="Dy_d_M_avg_Tc (uSec)") -> ("Tick Count(uSec)"=w487:u32)
  }
  n251 = for {
    N: w8 -> [_]
    tunnel: ["Dp_d_M_avg_Tc (uSec)"] -> w1
    tunnel: [w489] -> w7 mode=indexing
    tunnel: [w488] -> w6 mode=indexing
    n252 = local read "Encoder Position_p"() -> (w488:i32)
    n253 = call "Wait2"("Count(uSec)"="Dp_d_M_avg_Tc (uSec)") -> ("Tick Count(uSec)"=w489:u32)
  }
  n254 = while "Omega_y (Mavg)" {
    tunnel: w5 -> [w514]
    shift-right: [w512] -> _
    shift-left: w4 -> [w517]
    shift-right: [w511] -> _
    shift-left: w3 -> [w513]
    shift-right: [w506] -> _
    shift-left: _ -> [w510]
    tunnel: w2 -> [w505]
    stop <- FALSE stop-if-true
    w493 = fxp<+/-,32,0> 0.3183098859153688  # L/2/pi
    w502 = fxp<+,32,0> 0.1953125  # 800/4096
    w508 = fxp<+/-,27,3> 0.007853984832763672  # 2*pi/800
    n255 = call "Tick Count6"() -> ("Tick Count(uSec)"=w518:u32)
    n256 = Index Array(array=w517, index=0) -> (element=w516:u32)
    n257 = Index Array(array=w513, index=0) -> (element=w515:i32)
    n258 = Multiply(x=w514, y=w505) -> (x*y=w520:i32)
    n259 = Add(x=w520, y=w516) -> (x+y=w519:u32)
    n260 = Greater Or Equal?(x=w518, y=w519) -> (x >= y?=w509:bool)
    n261 = case shown="True" w509 {
      tunnel: w518 -> [_ w541]
      tunnel: w514 -> [_ w538]
      tunnel: w517 -> [w525 w540]
      tunnel: w516 -> [_ w539]
      tunnel: w515 -> [_ w535]
      tunnel: w513 -> [w524 w537]
      tunnel: [w523 w533] -> w506
      tunnel: [w525 w532] -> w512
      tunnel: [w524 w531] -> w511
      tunnel: w510 -> [w523 _]
      frame False {
      }
      frame True {
        # "count/s"
        n262 = local read "Encoder Position_y"() -> (w534:i32)
        n263 = Subtract(x=w541, y=w539) -> (x-y=w542:u32)
        n264 = Insert Into Array(array=w540, new element=w541) -> (w544:u32[])  [unwired: 1 in]
        n265 = Subtract(x=w534, y=w535) -> (x-y=w529:i32)
        n266 = Insert Into Array(array=w537, index=w538, new element=w534) -> (w545:i32[])
        n267 = To Fixed-Point(number=w542) -> (fixed-point=w528:fxp<+,32,32>)  [unwired: 1 in]
        n268 = To Fixed-Point(number=w529) -> (fixed-point=w536:fxp<+/-,32,32>)  [unwired: 1 in]
        n269 = Divide(x=w528, y=fxp<+,32,32> 1000000.0) -> (x/y=w527:fxp<+/-,64,32>)
        n270 = Delete From Array(array=w544, length=1, index=0) -> (array with subset deleted=w532:u32[])  [unwired: 1 out]
        n271 = Delete From Array(array=w545, length=1, index=0) -> (array with subset deleted=w531:i32[])  [unwired: 1 out]
        n272 = Divide(x=w536, y=w527) -> (x/y=w533:fxp<+/-,40,20>)
      }
    }
    n273 = local read "Mag. factor_p"() -> (w501:fxp<+/-,20,3>)
    n274 = local read "Mag. encoder_y"() -> (w504:bool)
    n275 = local read "Belt_in_y"() -> (w495:fxp<+/-,6,6>)
    n276 = Multiply(x=w508, y=w506) -> (x*y=w498:fxp<+/-,44,14>)
    n277 = Divide(x=w502, y=w501) -> (x/y=w500:fxp<+/-,32,1>)
    n278 = local read "Belt_out_y"() -> (w496:fxp<+/-,7,7>)
    n279 = Select(t=w500, s=w504, f=fxp<+/-,2,2> 1.0) -> (s? t:f=w499:fxp<+/-,33,2>)
    n280 = Multiply(x=w493, y=w495) -> (x*y=w494:fxp<+/-,38,6>)
    n281 = Multiply(x=w499, y=w498) -> (x*y=w497:fxp<+/-,36,14>)
    "omega_y (Mavg)" <- w497
    n282 = Divide(x=w494, y=w496) -> (x/y=w492:fxp<+/-,45,6>)
    n283 = Multiply(x=w492, y=w497) -> (x*y=→"Dy_d (Mavg)":fxp<+/-,36,14>)
  }
  n284 = while "Omega_p (Mavg)" {
    tunnel: w8 -> [w571]
    shift-right: [w569] -> _
    shift-left: w7 -> [w574]
    shift-right: [w568] -> _
    shift-left: w6 -> [w570]
    shift-right: [w567] -> _
    shift-left: _ -> [w566]
    tunnel: w1 -> [w564]
    stop <- FALSE stop-if-true
    w553 = fxp<+/-,27,3> 0.007853984832763672  # 2*pi/800
    w555 = fxp<+,32,0> 0.1953125  # 800/4096
    w552 = fxp<+/-,32,0> 0.3183098859153688  # L/2/pi
    n285 = call "Tick Count5"() -> ("Tick Count(uSec)"=w575:u32)
    n286 = Index Array(array=w574, index=0) -> (element=w573:u32)
    n287 = Index Array(array=w570, index=0) -> (element=w572:i32)
    n288 = Multiply(x=w571, y=w564) -> (x*y=w577:i32)
    n289 = Add(x=w577, y=w573) -> (x+y=w576:u32)
    n290 = Greater Or Equal?(x=w575, y=w576) -> (x >= y?=w565:bool)
    n291 = case shown="True" w565 {
      tunnel: w575 -> [_ w598]
      tunnel: w571 -> [_ w595]
      tunnel: w574 -> [w582 w597]
      tunnel: w573 -> [_ w596]
      tunnel: w572 -> [_ w592]
      tunnel: w570 -> [w581 w594]
      tunnel: [w580 w590] -> w567
      tunnel: [w582 w589] -> w569
      tunnel: [w581 w588] -> w568
      tunnel: w566 -> [w580 _]
      frame False {
      }
      frame True {
        n292 = local read "Encoder Position_p"() -> (w591:i32)
        n293 = Subtract(x=w598, y=w596) -> (x-y=w599:u32)
        n294 = Subtract(x=w591, y=w592) -> (x-y=w583:i32)
        n295 = Insert Into Array(array=w597, new element=w598) -> (w601:u32[])  [unwired: 1 in]
        n296 = Insert Into Array(array=w594, index=w595, new element=w591) -> (w602:i32[])
        n297 = To Fixed-Point(number=w599) -> (fixed-point=w585:fxp<+,32,32>)  [unwired: 1 in]
        n298 = To Fixed-Point(number=w583) -> (fixed-point=w593:fxp<+/-,32,32>)  [unwired: 1 in]
        n299 = Delete From Array(array=w601, length=1, index=0) -> (array with subset deleted=w589:u32[])  [unwired: 1 out]
        n300 = Delete From Array(array=w602, length=1, index=0) -> (array with subset deleted=w588:i32[])  [unwired: 1 out]
        n301 = Divide(x=w585, y=fxp<+,32,32> 1000000.0) -> (x/y=w586:fxp<+/-,64,32>)
        n302 = Divide(x=w593, y=w586) -> (x/y=w590:fxp<+/-,40,20>)
      }
    }
    n303 = local read "Mag. factor_p"() -> (w556:fxp<+/-,20,3>)
    n304 = local read "Mag. encoder_p"() -> (w563:bool)
    n305 = local read "Belt_in_p"() -> (w560:fxp<+/-,6,6>)
    n306 = Divide(x=w555, y=w556) -> (x/y=w554:fxp<+/-,32,1>)
    n307 = local read "Belt_out_p"() -> (w559:fxp<+/-,7,7>)
    n308 = Multiply(x=w553, y=w567) -> (x*y=w561:fxp<+/-,44,14>)
    n309 = Select(t=w554, s=w563, f=fxp<+/-,2,2> 1.0) -> (s? t:f=w548:fxp<+/-,33,2>)
    n310 = Multiply(x=w552, y=w560) -> (x*y=w558:fxp<+/-,38,6>)
    n311 = Multiply(x=w548, y=w561) -> (x*y=w551:fxp<+/-,36,14>)
    "omega_p (Mavg)" <- w551
    n312 = Divide(x=w558, y=w559) -> (x/y=w550:fxp<+/-,45,6>)
    n313 = Multiply(x=w550, y=w551) -> (x*y=→"Dp_d (Mavg)":fxp<+/-,36,14>)
  }
  n314 = while "Quadrature drive_p" {
    stop <- FALSE stop-if-true
    n315 = local read "omega_p (rad/s)"() -> (w611:fxp<+/-,36,13>)
    n316 = local read "Fp_PID"() -> (w607:fxp<+/-,36,16>)
    n317 = call "Oriental_step_motor_PKP225.vi"("F_Threshold"=fxp<+,12,12> 10.0, "dFmr"=fxp<+/-,25,15> 0.0, "omega"=w611, "Fmr"=w607) -> ("vq_F"=→"vq_p_F":fxp<+/-,20,5>, "vd_F"=→"vd_p_F":fxp<+/-,20,5>)  [unwired: 6 in]
  }
  n318 = while "PID force controller_p" {
    shift-right: [w622] -> _
    shift-left: _ -> [w621]
    stop <- FALSE stop-if-true
    n319 = local read "D_p(mm)"() -> (w616:fxp<+/-,32,7>)
    n320 = local read "Dpr_for"() -> (w617:fxp<+/-,22,7>)
    n321 = call "Tick Count7"() -> ("Tick Count(uSec)"=w622:u32)
    n322 = Subtract(x=w622, y=w621) -> (x-y=w620:u32)
    n323 = Subtract(x=w617, y=w616) -> (x-y=w615:fxp<+/-,33,8>)
    n324 = Multiply(x="Kp_p", y=w615) -> (x*y=→"Fp_PID":fxp<+/-,64,20>)
    n325 = Divide(x=u32 1000, y=w620) -> (x/y=→"PID (kHz)":fxp<+/-,20,7>)
  }
  n326 = while "All switch" {
    stop <- FALSE stop-if-true
    n327 = case shown="True" "Encoder reset" {
      frame False {
        n328 = local write "Encoder reset_p"(FALSE ("Encoder reset_p")) -> ()
        n329 = local write "Encoder reset_y"(FALSE ("Encoder reset_y")) -> ()
      }
      frame True {
        n330 = flat-sequence {
          frame #0 {
            n331 = local write "Encoder reset_p"(TRUE ("Encoder reset_p")) -> ()
          }
          frame #1 {
            n332 = local write "Encoder reset_y"(TRUE ("Encoder reset_y")) -> ()
            n333 = local write "Encoder reset_p"(FALSE ("Encoder reset_p")) -> ()
          }
          frame #2 {
            n334 = local write "Encoder reset_y"(FALSE ("Encoder reset_y")) -> ()
          }
        }
      }
    }
  }
  n335 = while "Encoder_y" {
    shift-right: [w669] -> _
    shift-left: _ -> [w661]
    shift-right: [w668] -> _
    shift-left: _ -> [w660]
    shift-right: [w659] -> _
    shift-left: _ -> [w657]
    shift-right: [w665] -> _
    shift-left: _ -> [w662]
    shift-right: [w664] -> _
    shift-left: _ -> [w663]
    shift-right: [w658] -> _
    shift-left: _ -> [w656]
    stop <- FALSE stop-if-true
    w646 = fxp<+/-,16,1> 0.0244140625  # 2*50/4096
    w651 = fxp<+/-,20,-5> 0.00048828125  # L/4096
    w654 = fxp<+/-,20,-5> 0.002499997615814209  # L/800
    w636 = fxp<+/-,16,1> 0.125  # 2*50/800
    n336 = xnode "FPGA I/O Node"() -> ("Mod7/DIO2"=w670:bool, "Mod7/DIO3"=w671:bool)  [unwired: 2 in, 2 out]
    n337 = xnode "FPGA I/O Node"() -> ("Mod7/DIO6"=w667:bool, "Mod7/DIO7"=w666:bool)  [unwired: 2 in, 2 out]
    n338 = local read "Encoder reset_y"() -> (w641:bool)
    n339 = call "encoder_sub.vi"("A_pre"=w661, "B_pre"=w660, "Encoder Position_pre"=w657, "A input"=w670, "Encoder Position Reset"="Encoder reset_y", "B input"=w671) -> ("A"=w669:bool, "B"=w668:bool, "Encoder Position (Counts)"=w659:i32)  [unwired: 19 in]
    "Encoder Position_y1" <- w659
    n340 = call "encoder_sub.vi"("A_pre"=w662, "B_pre"=w663, "Encoder Position_pre"=w656, "A input"=w667, "Encoder Position Reset"=w641, "B input"=w666) -> ("A"=w665:bool, "B"=w664:bool, "Encoder Position (Counts)"=w658:i32)  [unwired: 19 in]
    "Encoder Position_y2" <- w658
    n341 = local read "Belt_in_y"() -> (w649:fxp<+/-,6,6>)
    n342 = local read "Belt_in_y"() -> (w653:fxp<+/-,6,6>)
    n343 = local read "Belt_out_y"() -> (w647:fxp<+/-,7,7>)
    n344 = Divide(x=w651, y="Mag. factor_y") -> (x/y=w650:fxp<+/-,41,13>)
    n345 = local read "Belt_out_y"() -> (w652:fxp<+/-,7,7>)
    n346 = To Fixed-Point(number=w658) -> (fixed-point=w633:fxp<+/-,32,32>)  [unwired: 1 in]
    n347 = local read "Mag. factor_y"() -> (w645:fxp<+/-,20,3>)
    n348 = To Fixed-Point(number=w659) -> (fixed-point=w637:fxp<+/-,32,32>)  [unwired: 1 in]
    n349 = Multiply(x=w650, y=w649) -> (x*y=w648:fxp<+/-,46,18>)
    n350 = Multiply(x=w654, y=w653) -> (x*y=w655:fxp<+/-,26,1>)
    n351 = Divide(x=w648, y=w647) -> (x/y=w635:fxp<+/-,53,18>)
    n352 = Divide(x=w655, y=w652) -> (x/y=w639:fxp<+/-,33,1>)
    n353 = Divide(x=w646, y=w645) -> (x/y=w632:fxp<+/-,32,1>)
    n354 = Multiply(x=w635, y=w633) -> (x*y=→"D_y2":fxp<+/-,37,7>)
    n355 = Multiply(x=w637, y=w636) -> (x*y=→"rad_y1":fxp<+/-,33,20>)
    n356 = Multiply(x=w639, y=w637) -> (x*y=→"D_y1":fxp<+/-,32,7>)
    n357 = Multiply(x=w633, y=w632) -> (x*y=→"rad_y2":fxp<+/-,33,20>)
  }
  n358 = while "Omega_y(T method)" {
    shift-right: [w698] -> _
    shift-left: _ -> [w699]
    shift-right: [w675] -> _
    shift-left: _ -> [w701]
    shift-right: [w703] -> _
    shift-left: _ -> [w704]
    shift-right: [w691] -> _
    shift-left: _ -> [w689]
    shift-right: [w684] -> _
    shift-left: _ -> [w690]
    shift-right: [w687] -> _
    shift-left: _ -> [w688]
    stop <- FALSE stop-if-true
    w682 = fxp<+/-,32,0> 0.3183098859153688  # L/2/pi
    w693 = fxp<+,32,0> 0.1953125  # 800/4096
    w697 = fxp<+/-,32,0> 0.3183098859153688  # L/2/pi
    n359 = local read "Encoder Position_y1"() -> (w698:i32)
    n360 = call "Tick Count2"() -> ("Tick Count(Ticks)"=w685:u32)
    n361 = local read "Encoder Position_y2"() -> (w691:i32)
    n362 = local read "Mag. factor_y"() -> (w692:fxp<+/-,20,3>)
    n363 = call "omega_sub_Encoder_800ppr.vi"("mt0"="mt0_omega_y", "omega_pre"=w701, "ticks_m_pre"=w704, "ticks"=w685, "count_pre"=w699, "count"=w698) -> ("ticks_m"=w703:u32, "mt"=→"mt_omega_y1":u32, "omega"=w675:fxp<+/-,36,13>)  [unwired: 3 in]
    "omega_y1 (T)" <- w675
    n364 = call "omega_sub_Encoder_800ppr.vi"("omega_pre"=w690, "ticks_m_pre"=w688, "ticks"=w685, "count_pre"=w689, "count"=w691) -> ("ticks_m"=w687:u32, "mt"=→"mt_omega_y2":u32, "omega"=w684:fxp<+/-,36,13>)  [unwired: 4 in]
    n365 = local read "Belt_in_y"() -> (w681:fxp<+/-,6,6>)
    n366 = local read "Belt_out_y"() -> (w679:fxp<+/-,7,7>)
    n367 = Divide(x=w693, y=w692) -> (x/y=w683:fxp<+/-,32,1>)
    n368 = Multiply(x=w697, y="Belt_in_y") -> (x*y=w695:fxp<+/-,38,6>)
    n369 = Multiply(x=w682, y=w681) -> (x*y=w680:fxp<+/-,38,6>)
    n370 = Divide(x=w680, y=w679) -> (x/y=w673:fxp<+/-,45,6>)
    n371 = Divide(x=w695, y="Belt_out_y") -> (x/y=w676:fxp<+/-,20,1>)
    n372 = Multiply(x=w684, y=w683) -> (x*y=w672:fxp<+/-,36,13>)
    "omega_y2 (T)" <- w672
    n373 = Multiply(x=w676, y=w675) -> (x*y=→"Dy1_d (T)":fxp<+/-,36,13>)
    n374 = Multiply(x=w673, y=w672) -> (x*y=→"Dy2_d (T)":fxp<+/-,36,13>)
  }
  n375 = while {
    stop <- FALSE stop-if-true
    n376 = case shown="True" "Set 3" {
      frame False {
      }
      frame True {
        n377 = local write "Kp_p"(fxp<+/-,36,9> 100.0 ("Kp_p")) -> ()
        n378 = local write item#-1(fxp<+,22,6> 3.0 ("fp_tolorance")) -> ()
      }
    }
    n379 = case shown="True" "Set 2" {
      frame False {
      }
      frame True {
        n380 = local write "Kp_p"(fxp<+/-,36,9> 50.0 ("Kp_p")) -> ()
        n381 = local write item#-1(fxp<+,22,6> 1.5 ("fp_tolorance")) -> ()
      }
    }
    n382 = case shown="True" "Set 1" {
      frame False {
      }
      frame True {
        n383 = local write "Kp_p"(fxp<+/-,36,9> 50.0 ("Kp_p")) -> ()
        n384 = local write item#-1(fxp<+,22,6> 3.0 ("fp_tolorance")) -> ()
      }
    }
    n385 = case shown="True" "Set 5" {
      frame False {
      }
      frame True {
        n386 = local write "Kp_p"(fxp<+/-,36,9> 150.0 ("Kp_p")) -> ()
        n387 = local write item#-1(fxp<+,22,6> 3.0 ("fp_tolorance")) -> ()
      }
    }
    n388 = case shown="True" "Set 6" {
      frame False {
      }
      frame True {
        n389 = local write "Kp_p"(fxp<+/-,36,9> 150.0 ("Kp_p")) -> ()
        n390 = local write item#-1(fxp<+,22,6> 1.5 ("fp_tolorance")) -> ()
      }
    }
    n391 = case shown="True" "Set 4" {
      frame False {
      }
      frame True {
        n392 = local write "Kp_p"(fxp<+/-,36,9> 100.0 ("Kp_p")) -> ()
        n393 = local write item#-1(fxp<+,22,6> 1.5 ("fp_tolorance")) -> ()
      }
    }
  }
  n394 = while {
    stop <- FALSE stop-if-true
    n395 = local read "omega_p (Mavg)"() -> (w727:fxp<+/-,36,14>)
    n396 = xnode "Butterworth Filter"("input data"=w727, "scaled coefficients"="scaled coefficients") -> ("output data"=→"omega_p (Mavg w. f)":fxp<+/-,36,18>)  [unwired: 1 in]
  }
